vi "Draw Tree Control.vi"(8 "error in (no error)":errorcluster, 11 "File Explorer in":refnum<class "File Explorer.lvclass">) -> (0 "error out":errorcluster, 3 "File Explorer out":refnum<class "File Explorer.lvclass">)   [LabVIEW 2020, in "File Explorer.lvlib" / "File Explorer.lvclass"]
uses:
  <vilib>/gpm_packages/@cs/file-explorer-extension/Source/File Explorer/File Explorer/File Explorer.lvclass
  <vilib>/gpm_packages/@cs/file-explorer-extension/Source/File Explorer/File Explorer/File Explorer.lvclass/File Explorer.ctl
  <vilib>/picture/picture.llb/imagedata.ctl
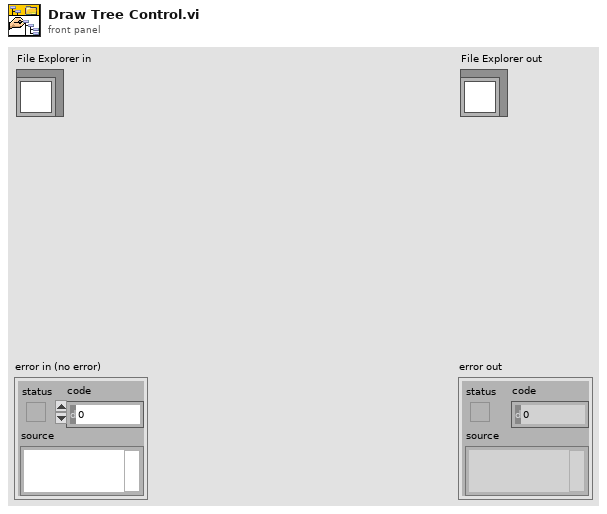
[diagram p1: front panel]
types:
  T1 = typedef "imagedata.ctl" = cluster{"image type":i32, "image depth":i32, "image":u8[], "mask":u8[], "colors":u32[], "Rectangle":cluster{"left":i16, "top":i16, "right":i16, "bottom":i16}}
  T2 = cluster{"Left Cell String":string, "Child Text":string[], "Child Tag":string, "Item Indent":i32, "Child Only?":bool, "Glyph Index":i32}[]
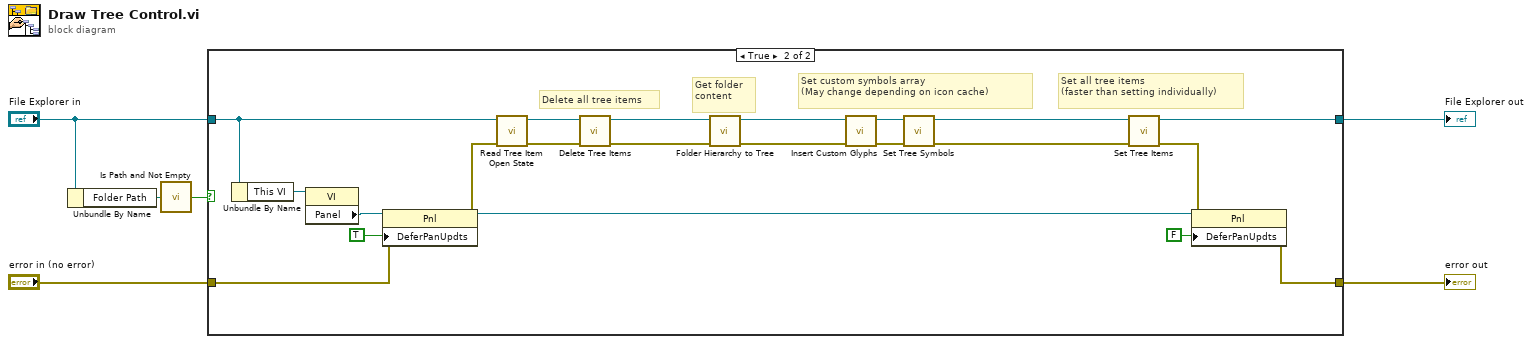
[diagram p0: block diagram]
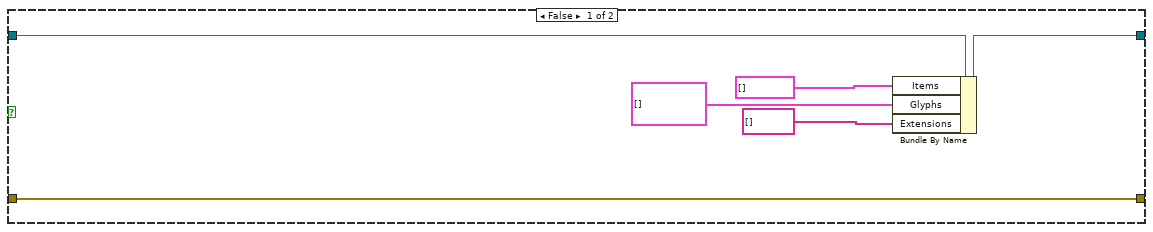
[diagram p2: hidden frame]
diagram:
  n1 = Unbundle By Name("File Explorer in") -> ("Folder Path"=w6:path)
  n2 = call <vilib>:"Is Path and Not Empty.vi"("path"=w6) -> ("Is Path and Not Empty?"=w5:bool)  [unwired: 4 in]
  n3 = case shown="True" w5 {
    tunnel: [w12 w13] -> w3
    tunnel: "error in (no error)" -> [w12 w18]
    tunnel: [w10 w30] -> w1
    tunnel: "File Explorer in" -> [w11 w22]
    frame False {
      n4 = Bundle By Name(cluster=w11, "Items"=T2 [], "Glyphs"=T1[] [], "Extensions"=string[] []) -> (w10:refnum<class "File Explorer.lvclass">)
    }
    frame True {
      # "Set all tree items\n(faster than setting individually)"
      # "Set custom symbols array\n(May change depending on icon cache)"
      # "Get folder\ncontent"
      # "Delete all tree items"
      n5 = Unbundle By Name(w22) -> ("This VI"=w21:refnum<vi>)
      n6 = property class="VI"(reference=w21) -> ("Panel"=w20:refnum<vi>)  [unwired: 1 in, 2 out]
      n7 = property class="Pnl"(reference=w20, error in=w18, "DeferPanUpdts"=TRUE ("Defer Panel Updates")) -> (reference out=w15:refnum<vi>, error out=w17:errorcluster)
      n8 = call <vilib>:"Read Tree Item Open State.vi"("error in (no error)"=w17, "File Explorer in"=w22) -> ("error out"=w23:errorcluster, "File Explorer out"=w24:refnum<class "File Explorer.lvclass">)  [unwired: 8 in]
      n9 = call <vilib>:"Delete Tree Items.vi"("error in (no error)"=w23, "File Explorer in"=w24) -> ("error out"=w33:errorcluster, "File Explorer out"=w26:refnum<class "File Explorer.lvclass">)  [unwired: 8 in]
      n10 = call <vilib>:"Folder Hierarchy to Tree.vi"("error in (no error)"=w33, "File Explorer in"=w26) -> ("error out"=w27:errorcluster, "File Explorer out"=w25:refnum<class "File Explorer.lvclass">)  [unwired: 8 in]
      n11 = call <vilib>:"Insert Custom Glyphs.vi"("error in (no error)"=w27, "File Explorer in"=w25) -> ("error out"=w28:errorcluster, "File Explorer out"=w32:refnum<class "File Explorer.lvclass">)  [unwired: 8 in]
      n12 = call <vilib>:"Set Tree Symbols.vi"("error in (no error)"=w28, "File Explorer in"=w32) -> ("error out"=w29:errorcluster, "File Explorer out"=w31:refnum<class "File Explorer.lvclass">)  [unwired: 8 in]
      n13 = call <vilib>:"Set Tree Items.vi"("error in (no error)"=w29, "File Explorer in"=w31) -> ("error out"=w14:errorcluster, "File Explorer out"=w30:refnum<class "File Explorer.lvclass">)  [unwired: 8 in]
      n14 = property class="Pnl"(reference=w15, error in=w14, "DeferPanUpdts"=FALSE ("Defer Panel Updates")) -> (error out=w13:errorcluster)  [unwired: 1 out]
    }
  }
  "error out" <- w3
  "File Explorer out" <- w1
